vi "GetAttributeViBoolean_SA-HD_OB.vi"(8 "error in (no error)":errorcluster {"code" format="%.0x"}, 9 "AttributeID":u32(ring)=1150457 items=["SA_HARMONICDISTORTION_AVERAGE_ENABLED"=1150457, "SA_HARMONICDISTORTION_FUNDAMENTAL_FREQUENCY_AUTO_ENABLED"=1150461, "SA_HARMONICDISTORTION_RANGETABLE_ENABLED"=1150472, "SA_HARMONICDISTORTION_SWEEPCOUPLING_RESOLUTION_BANDWIDTH_AUTO_ENABLED"=1150465, "SA_HARMONICDISTORTION_SWEEPCOUPLING_SWEEP_TIME_AUTO_ENABLED"=1150467, "SA_HARMONICDISTORTION_SWEEPCOUPLING_VIDEO_BANDWIDTH_AUTO_ENABLED"=1150469, "SA_OCCUPIEDBANDWIDTH_AVERAGE_ENABLED"=1150290, "SA_OCCUPIEDBANDWIDTH_DETECTOR_TYPE_AUTO_ENABLED"=1150287, "SA_OCCUPIEDBANDWIDTH_DISPLAY_WINDOWY_AUTO_SCALE_ENABLED"=1150308, "SA_OCCUPIEDBANDWIDTH_DISPLAY_XDB_BOUNDARIES_ENABLED"=1150870, "SA_OCCUPIEDBANDWIDTH_IF_GAIN_AUTO_ENABLED"=1150662, "SA_OCCUPIEDBANDWIDTH_IF_GAIN"=1150661, "SA_OCCUPIEDBANDWIDTH_LIMIT_TEST_ENABLED"=1150332, "SA_OCCUPIEDBANDWIDTH_MARKER_COUPLE_ENABLED"=1150324, "SA_OCCUPIEDBANDWIDTH_MARKER_ENABLED"=1150326, "SA_OCCUPIEDBANDWIDTH_MARKER_MAX_HOLD_ENABLED"=1150209, "SA_OCCUPIEDBANDWIDTH_SWEEPCOUPLING_RESOLUTION_BANDWIDTH_AUTO_ENABLED"=1150295, "SA_OCCUPIEDBANDWIDTH_SWEEPCOUPLING_SWEEP_TIME_AUTO_ENABLED"=1150292, "SA_OCCUPIEDBANDWIDTH_SWEEPCOUPLING_VIDEO_BANDWIDTH_AUTO_ENABLED"=1150297], 11 "instrument handle":refnum<k15>) -> (0 "error out":errorcluster {"code" format="%.0x"}, 2 "AttributeValue":bool, 3 "instrument handle out":refnum<k15>)   [LabVIEW 2009, in "Keysight XSAn.lvlib"]
doc: "Gets a Boolean attribute from the instrument driver.\nThe following Attributes are supported:\n\nSA_HARMONICDISTORTION_AVERAGE_ENABLED\nSA_HARMONICDISTORTION_FUNDAMENTAL_FREQUENCY_AUTO_ENABLED\nSA_HARMONICDISTORTION_RANGETABLE_ENABLED\nSA_HARMONICDISTORTION_SWEEPCOUPLING_RESOLUTION_BANDWIDTH_AUTO_ENABLED\nSA_HARMONICDISTORTION_SWEEPCOUPLING_SWEEP_TIME_AUTO_ENABLED\nSA_HARMONICDISTORTION_SWEEPCOUPLING_VIDEO_BANDWIDTH_AUTO_ENABLED\nSA_OCCUPIEDBANDWIDTH_AVERAGE_ENABLED\nSA_OCCUPIEDBANDWIDTH_DETECTOR_TYPE_AUTO_ENABLED\nSA_OCCUPIEDBANDWIDTH_DISPLAY_WINDOWY_AUTO_SCALE_ENABLED\nSA_OCCUPIEDBANDWIDTH_DISPLAY_XDB_BOUNDARIES_ENABLED\nSA_OCCUPIEDBANDWIDTH_IF_GAIN_AUTO_ENABLED\nSA_OCCUPIEDBANDWIDTH_IF_GAIN\nSA_OCCUPIEDBANDWIDTH_LIMIT_TEST_ENABLED\nSA_OCCUPIEDBANDWIDTH_MARKER_COUPLE_ENABLED\nSA_OCCUPIEDBANDWIDTH_MARKER_ENABLED\nSA_OCCUPIEDBANDWIDTH_MARKER_MAX_HOLD_ENABLED\nSA_OCCUPIEDBANDWIDTH_SWEEPCOUPLING_RESOLUTION_BANDWIDTH_AUTO_ENABLED\nSA_OCCUPIEDBANDWIDTH_SWEEPCOUPLING_SWEEP_TIME_AUTO_ENABLED\nSA_OCCUPIEDBANDWIDTH_SWEEPCOUPLING_VIDEO_BANDWIDTH_AUTO_ENABLED"
uses:
  <instrlib>/Keysight XSAn/Keysight XSAn.lvlib
  AgXSAn.dll
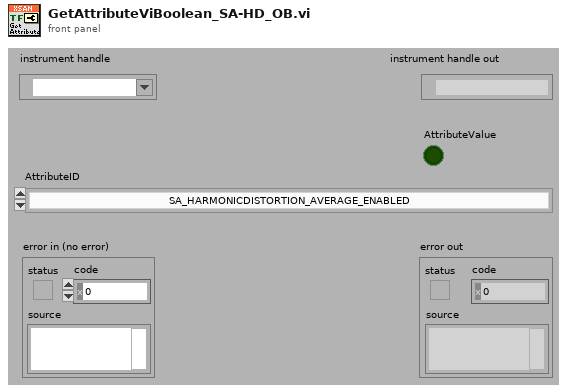
[diagram p1: front panel]
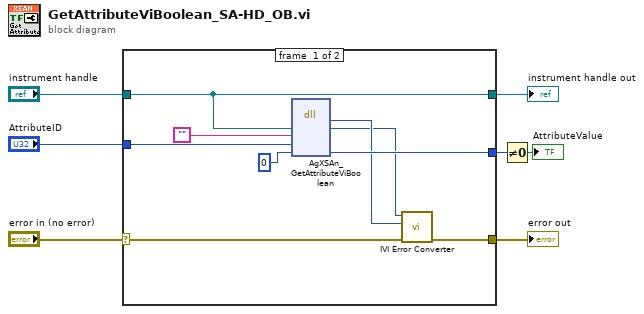
[diagram p0: block diagram]
diagram:
  n1 = case shown="No Error" "error in (no error)" {
    selector: "error in (no error)" -> [w16 w18]
    tunnel: [w15 w18] -> w7
    tunnel: "instrument handle" -> [w11 w17]
    tunnel: "AttributeID" -> [w14 _]
    tunnel: [w12 _] -> w2
    tunnel: [w11 w17] -> w1
    frame #0 {
      n2 = dll-call lib="AgXSAn**.dll" fn="AgXSAn_GetAttributeViBoolean"("Vi"=w11, "RepCapIdentifier"="", "AttributeID"=w14, "AttributeValue"=i16 0) -> ("return type"=w9:i32, "Vi"=w8:u32, "AttributeValue"=w12:i16)  [unwired: 5 in, 2 out]
      n3 = call <instrlib>:"IVI Error Converter.vi"("error in (no error)"=w16, "IVI error code (0)"=w9, "instrument handle"=w8) -> ("error out"=w15:errorcluster)  [unwired: 7 in, 1 out]
    }
    frame #1 {
    }
  }
  "error out" <- w7
  "instrument handle out" <- w1
  n4 = Not Equal To 0?(x=w2) -> (x != 0?=→"AttributeValue":bool)
